vi "Func-엑셀 데이터를 그래프로 출력.vi"() -> ()   [LabVIEW 2015] (continued)
50.927\n45\t45\t50.93\n45\t45\t50.93\n45\t45\t50.933\n45\t45\t50.933\n45\t45\t50.934\n45\t45\t50.935\n45\t45\t50.93\n45\t45\t50.929\n45\t45\t50.927\n45\t45\t50.927\n45\t45\t50.927\n45\t45\t50.926\n45\t45\t50.929\n45\t45\t50.935\n45\t45\t50.938\n45\t45\t50.937\n45\t45\t50.939\n45\t45\t50.942\n45\t45\t50.94\n45\t45\t50.939\n45\t45\t50.937\n45\t45\t50.945\n45\t45\t50.944\n45\t45\t50.944\n45\t45\t50.949\n45\t45\t50.95\n45\t45\t50.952\n45\t45\t50.949\n45\t45\t50.95\n45\t45\t50.949\n45\t45\t50.95\n45\t45\t50.95\n45\t45\t50.95\n45.083\t45.06\t51.454\n45.167\t45.12\t51.454\n45.25\t44.98\t51.464\n45.333\t44.93\t51.459\n45.417\t44.88\t51.464\n45.5\t44.82\t51.465\n45.583\t44.73\t51.473\n45.667\t44.67\t51.468\n45.75\t44.61\t51.472\n45.833\t44.54\t51.482\n45.917\t44.49\t51.481\n46\t44.45\t51.484\n46.083\t44.44\t51.485\n46.167\t44.44\t51.489\n46.25\t44.46\t51.483\n46.333\t44.51\t51.48\n46.417\t44.56\t51.492\n46.5\t44.64\t51.481\n46.583\t44.72\t51.489\n46.667\t44.81\t51.487\n46.75\t44.91\t51.487\n46.833\t45.01\t51.496\n46.917\t45.11\t51.491\n47\t45.22\t51.492\n47.083\t45.34\t51.484\n47.167\t45.46\t51.488\n47.25\t45.57\t51.495\n47.333\t45.67\t51.494\n47.417\t45.78\t51.486\n47.5\t45.88\t51.496\n47.583\t45.98\t51.486\n47.667\t46.07\t51.493\n47.75\t46.16\t51.49\n47.833\t46.25\t51.499\n47.917\t46.34\t51.495\n48\t46.42\t51.504\n48.083\t46.51\t51.499\n48.167\t46.59\t51.522\n48.25\t46.67\t51.518\n48.333\t46.77\t51.516\n48.417\t46.84\t51.523\n48.5\t46.93\t51.53\n48.583\t47.01\t51.538\n48.667\t47.1\t51.536\n48.75\t47.17\t51.552\n48.833\t47.24\t51.558\n48.917\t47.32\t51.562\n49\t47.4\t51.574\n49.083\t47.48\t51.588\n49.167\t47.55\t51.587\n49.25\t47.63\t51.607\n49.333\t47.71\t51.613\n49.417\t47.79\t51.635\n49.5\t47.87\t51.639\n49.583\t47.95\t51.655\n49.667\t48.03\t51.664\n49.75\t48.11\t51.681\n49.833\t48.18\t51.702\n49.917\t48.27\t51.708\n50\t48.35\t51.731\n50.083\t48.43\t51.746\n50.167\t48.52\t51.762\n50.25\t48.61\t51.783\n50.333\t48.69\t51.804\n50.417\t48.78\t51.823\n50.5\t48.86\t51.837\n50.583\t48.95\t51.854\n50.667\t49.02\t51.886\n50.75\t49.11\t51.9\n50.833\t49.19\t51.919\n50.917\t49.28\t51.943\n51\t49.35\t51.965\n51.083\t49.43\t51.987\n51.167\t49.52\t52.009\n51.25\t49.61\t52.038\n51.333\t49.68\t52.061\n51.417\t49.76\t52.08\n51.5\t49.83\t52.113\n51.583\t49.91\t52.137\n51.667\t49.99\t52.161\n51.75\t50.07\t52.2\n51.833\t50.15\t52.221\n51.917\t50.23\t52.246\n52\t50.31\t52.281\n52.083\t50.39\t52.312\n52.167\t50.49\t52.343\n52.25\t50.57\t52.374\n52.333\t50.65\t52.403\n52.417\t50.73\t52.438\n52.5\t50.82\t52.46\n52.583\t50.89\t52.497\n52.667\t50.98\t52.536\n52.75\t51.07\t52.575\n52.833\t51.16\t52.593\n52.917\t51.24\t52.629\n53\t51.32\t52.674\n53.083\t51.4\t52.711\n53.167\t51.48\t52.737\n53.25\t51.57\t52.782\n53.333\t51.66\t52.818\n53.417\t51.74\t52.858\n53.5\t51.82\t52.893\n53.583\t51.89\t52.931\n53.667\t51.97\t52.97\n53.75\t52.05\t53.007\n53.833\t52.14\t53.043\n53.917\t52.22\t53.093\n54\t52.3\t53.124\n54.083\t52.38\t53.176\n54.167\t52.47\t53.209\n54.25\t52.54\t53.245\n54.333\t52.64\t53.289\n54.417\t52.72\t53.343\n54.5\t52.79\t53.374\n54.583\t52.86\t53.423\n54.667\t52.94\t53.472\n54.75\t53.03\t53.514\n54.833\t53.11\t53.549\n54.917\t53.2\t53.603\n55\t53.28\t53.643\n55.083\t53.37\t53.687\n55.167\t53.44\t53.737\n55.25\t53.52\t53.783\n55.333\t53.61\t53.831\n55.417\t53.7\t53.877\n55.5\t53.78\t53.917\n55.583\t53.86\t53.972\n55.667\t53.93\t54.016\n55.75\t54.02\t54.066\n55.833\t54.1\t54.117\n55.917\t54.18\t54.164\n56\t54.27\t54.219\n56.083\t54.34\t54.265\n56.167\t54.42\t54.307\n56.25\t54.5\t54.362\n56.333\t54.58\t54.414\n56.417\t54.66\t54.463\n56.5\t54.73\t54.522\n56.583\t54.79\t54.571\n56.667\t54.88\t54.629\n56.75\t54.96\t54.674\n56.833\t55.03\t54.72\n56.917\t55.1\t54.784\n57\t55.19\t54.833\n57.083\t55.26\t54.886\n57.167\t55.34\t54.939\n57.25\t55.41\t54.992\n57.333\t55.49\t55.051\n57.417\t55.58\t55.099\n57.5\t55.66\t55.154\n57.583\t55.75\t55.209\n57.667\t55.82\t55.265\n57.75\t55.91\t55.312\n57.833\t55.99\t55.375\n57.917\t56.07\t55.438\n58\t56.16\t55.492\n58.083\t56.24\t55.546\n58.167\t56.31\t55.595\n58.25\t56.38\t55.664\n58.333\t56.47\t55.716\n58.417\t56.56\t55.777\n58.5\t56.65\t55.834\n58.583\t56.73\t55.902\n58.667\t56.8\t55.946\n58.75\t56.88\t56.002\n58.833\t56.96\t56.062\n58.917\t57.06\t56.121\n59\t57.15\t56.189\n59.083\t57.22\t56.238\n59.167\t57.3\t56.307\n59.25\t57.38\t56.354\n59.333\t57.46\t56.419\n59.417\t57.53\t56.482\n59.5\t57.61\t56.538\n59.583\t57.69\t56.598\n59.667\t57.77\t56.665\n59.75\t57.86\t56.718\n59.833\t57.94\t56.78\n59.917\t58.02\t56.843\n60\t58.1\t56.904\n60.083\t58.18\t56.961\n60.167\t58.26\t57.021\n60.25\t58.35\t57.083\n60.333\t58.43\t57.157\n60.417\t58.51\t57.206\n60.5\t58.59\t57.264\n60.583\t58.66\t57.339\n60.667\t58.75\t57.397\n60.75\t58.84\t57.464\n60.833\t58.93\t57.522\n60.917\t59.02\t57.582\n61\t59.1\t57.652\n61.083\t59.19\t57.711\n61.167\t59.27\t57.785\n61.25\t59.35\t57.839\n61.333\t59.45\t57.91\n61.417\t59.53\t57.975\n61.5\t59.62\t58.027\n61.583\t59.72\t58.096\n61.667\t59.8\t58.163\n61.75\t59.89\t58.225\n61.833\t59.97\t58.293\n61.917\t60.05\t58.357\n62\t60.14\t58.418\n62.083\t60.22\t58.486\n62.167\t60.3\t58.55\n62.25\t60.37\t58.618\n62.333\t60.45\t58.689\n62.417\t60.53\t58.754\n62.5\t60.6\t58.819\n62.583\t60.69\t58.891\n62.667\t60.76\t58.95\n62.75\t60.84\t59.013\n62.833\t60.92\t59.083\n62.917\t61.01\t59.146\n63\t61.09\t59.214\n63.083\t61.18\t59.285\n63.167\t61.27\t59.348\n63.25\t61.35\t59.42\n63.333\t61.42\t59.478\n63.417\t61.51\t59.56\n63.5\t61.59\t59.621\n63.583\t61.68\t59.683\n63.667\t61.75\t59.76\n63.75\t61.84\t59.826\n63.833\t61.91\t59.893\n63.917\t62\t59.955\n64\t62.07\t60.034\n64.083\t62.15\t60.115\n64.167\t62.21\t60.175\n64.25\t62.3\t60.236\n64.333\t62.39\t60.311\n64.417\t62.47\t60.374\n64.5\t62.56\t60.449\n64.583\t62.65\t60.524\n64.667\t62.74\t60.598\n64.75\t62.83\t60.652\n64.833\t62.9\t60.731\n65\t62.97\t60.794\n65\t62.98\t60.795\n65\t62.99\t60.803\n65\t63\t60.809\n65\t63.01\t60.811\n65\t63.02\t60.817\n65\t63.04\t60.828\n65\t63.05\t60.836\n65\t63.05\t60.841\n65\t63.06\t60.851\n65\t63.07\t60.861\n65\t63.07\t60.867\n65\t63.08\t60.875\n65\t63.09\t60.88\n65\t63.11\t60.889\n65\t63.12\t60.898\n65\t63.13\t60.905\n65\t63.14\t60.909\n65\t63.15\t60.914\n65\t63.15\t60.922\n65\t63.16\t60.93\n65\t63.16\t60.938\n65\t63.17\t60.946\n65\t63.17\t60.953\n65\t63.18\t60.964\n65\t63.19\t60.971\n65\t63.2\t60.98\n65\t63.21\t60.988\n65\t63.22\t60.994\n65\t63.22\t61.006\n65\t63.24\t61.009\n65\t63.25\t61.012\n65\t63.26\t61.018\n65\t63.27\t61.022\n65\t63.27\t61.024\n65\t63.27\t61.031\n65\t63.28\t61.039\n65\t63.28\t61.048\n65\t63.29\t61.056\n65\t63.3\t61.064\n65\t63.31\t61.069\n65\t63.32\t61.078\n65\t63.33\t61.082\n65\t63.34\t61.088\n65\t63.35\t61.096\n65\t63.35\t61.102\n65\t63.36\t61.114\n65\t63.36\t61.121\n65\t63.37\t61.123\n65\t63.37\t61.136\n65\t63.37\t61.141\n65\t63.38\t61.146\n65\t63.39\t61.153\n65\t63.4\t61.16\n65\t63.4\t61.173\n65\t63.41\t61.178\n65\t63.42\t61.186\n65\t63.43\t61.193\n65\t63.44\t61.202\n65\t63.45\t61.209\n65\t63.45\t61.213\n65\t63.46\t61.222\n65\t63.47\t61.228\n65\t63.47\t61.234\n65\t63.47\t61.238\n65\t63.48\t61.246\n65\t63.49\t61.252\n65\t63.5\t61.26\n65\t63.51\t61.268\n65\t63.52\t61.28\n65\t63.53\t61.288\n65\t63.53\t61.292\n65\t63.54\t61.305\n65\t63.55\t61.307\n65\t63.55\t61.314\n65\t63.56\t61.32\n65\t63.57\t61.327\n65\t63.57\t61.33\n65\t63.57\t61.336\n65\t63.58\t61.346\n65\t63.59\t61.35\n65\t63.59\t61.357\n65\t63.6\t61.363\n65\t63.61\t61.375\n65\t63.61\t61.381\n65\t63.62\t61.387\n65\t63.63\t61.395\n65\t63.64\t61.401\n65\t63.64\t61.41\n65\t63.65\t61.416\n65\t63.66\t61.423\n65\t63.66\t61.429\n65\t63.67\t61.439\n65\t63.67\t61.449\n65\t63.67\t61.45\n65\t63.67\t61.455\n65\t63.68\t61.463\n65\t63.69\t61.469\n65\t63.69\t61.472\n65\t63.7\t61.477\n65\t63.71\t61.489\n65\t63.71\t61.498\n65\t63.72\t61.507\n65\t63.73\t61.509\n65\t63.74\t61.521\n65\t63.74\t61.525\n65\t63.75\t61.53\n65\t63.75\t61.535\n65\t63.76\t61.537\n65\t63.76\t61.549\n65\t63.77\t61.554\n65\t63.77\t61.56\n65\t63.77\t61.568\n65\t63.78\t61.577\n65\t63.79\t61.588\n65\t63.79\t61.605\n65\t63.8\t61.611\n65\t63.81\t61.618\n65\t63.81\t61.629\n65\t63.82\t61.635\n65\t63.83\t61.639\n65\t63.83\t61.642\n65\t63.84\t61.65\n65\t63.84\t61.654\n65\t63.85\t61.659\n65\t63.86\t61.666\n65\t63.86\t61.671\n65\t63.87\t61.679\n65\t63.87\t61.682\n65\t63.87\t61.689\n65\t63.88\t61.7\n65\t63.88\t61.709\n65\t63.89\t61.717\n65\t63.9\t61.727\n65\t63.9\t61.732\n65\t63.91\t61.739\n65\t63.91\t61.745\n65\t63.92\t61.75\n65\t63.92\t61.762\n65\t63.93\t61.763\n65\t63.93\t61.771\n65\t63.93\t61.782\n65\t63.93\t61.788\n65\t63.94\t61.795\n65\t63.94\t61.799\n65\t63.95\t61.812\n65\t63.96\t61.818\n65\t63.96\t61.827\n65\t63.97\t61.836\n65\t63.97\t61.844\n65\t63.98\t61.856\n65\t63.98\t61.862\n65\t63.98\t61.871\n65\t63.98\t61.878\n65\t63.99\t61.884\n65\t63.99\t61.889\n65\t64\t61.894\n65\t64.01\t61.898\n65\t64.01\t61.902\n65\t64.01\t61.912\n65\t64.02\t61.914\n65\t64.02\t61.922\n65\t64.03\t61.926\n65\t64.04\t61.931\n65\t64.05\t61.939\n65\t64.05\t61.948\n65\t64.06\t61.957\n65\t64.06\t61.966\n65\t64.07\t61.973\n65\t64.07\t61.982\n65\t64.08\t61.996\n65\t64.08\t62.001\n65\t64.08\t62.004\n65\t64.09\t62.016\n65\t64.1\t62.024\n65\t64.11\t62.028\n65\t64.12\t62.03\n65\t64.13\t62.035\n65\t64.13\t62.04\n65\t64.14\t62.046\n65\t64.15\t62.052\n65\t64.15\t62.062\n65\t64.16\t62.068\n65\t64.16\t62.077\n65\t64.17\t62.091\n65\t64.17\t62.094\n65\t64.18\t62.098\n65\t64.18\t62.109\n65\t64.18\t62.117\n65\t64.19\t62.121\n65\t64.19\t62.129\n65\t64.2\t62.136\n65\t64.2\t62.146\n65\t64.21\t62.152\n65\t64.21\t62.157\n65\t64.22\t62.162\n65\t64.22\t62.17\n65\t64.23\t62.176\n65\t64.23\t62.175\n65\t64.23\t62.183\n65\t64.24\t62.187\n65\t64.24\t62.195\n65\t64.24\t62.202\n65\t64.25\t62.211\n65\t64.25\t62.227\n65\t64.26\t62.232\n65\t64.26\t62.243\n65\t64.27\t62.257\n65\t64.27\t62.263\n65\t64.27\t62.268\n65\t64.28\t62.275\n65\t64.28\t62.283\n65\t64.28\t62.289\n65\t64.28\t62.296\n65\t64.29\t62.301\n65\t64.29\t62.306\n65\t64.3\t62.316\n65\t64.3\t62.325\n65\t64.31\t62.331\n65\t64.31\t62.339\n65\t64.32\t62.346\n65\t64.33\t62.353\n65\t64.33\t62.36\n65\t64.34\t62.359\n65\t64.34\t62.368\n65\t64.35\t62.374\n65\t64.35\t62.38\n65\t64.36\t62.39\n65\t64.36\t62.397\n65\t64.37\t62.405\n65\t64.37\t62.412\n65\t64.38\t62.419\n65\t64.38\t62.424\n65\t64.38\t62.43\n65\t64.38\t62.436\n65\t64.39\t62.443\n65\t64.39\t62.454\n65\t64.4\t62.459\n65\t64.4\t62.467\n65\t64.4\t62.475\n65\t64.41\t62.484\n65\t64.41\t62.491\n65\t64.42\t62.499\n65\t64.42\t62.505\n65\t64.42\t62.51\n65\t64.43\t62.521\n65\t64.44\t62.526\n65\t64.44\t62.534\n65\t64.45\t62.539\n65\t64.45\t62.545\n65\t64.45\t62.556\n65\t64.46\t62.563\n65\t64.46\t62.566\n65\t64.47\t62.575\n65\t64.47\t62.582\n65\t64.48\t62.591\n65\t64.48\t62.597\n65\t64.48\t62.602\n65\t64.49\t62.61\n65\t64.49\t62.62\n65\t64.5\t62.629\n65\t64.5\t62.632\n65\t64.51\t62.642\n65\t64.52\t62.649\n65\t64.52\t62.657\n65\t64.53\t62.662\n65\t64.53\t62.664\n65\t64.53\t62.673\n65\t64.54\t62.682\n65\t64.54\t62.689\n65\t64.55\t62.698\n65\t64.55\t62.705\n65\t64.56\t62.713\n65\t64.56\t62.718\n65\t64.57\t62.723\n65\t64.57\t62.729\n65\t64.57\t62.737\n65\t64.58\t62.74\n65\t64.58\t62.745\n65\t64.58\t62.758\n65\t64.59\t62.766\n65\t64.59\t62.769\n65\t64.59\t62.774\n65\t64.59\t62.784\n65\t64.59\t62.792\n65\t64.6\t62.798\n65\t64.6\t62.804\n65\t64.61\t62.82\n65\t64.61\t62.823\n65\t64.61\t62.827\n65\t64.62\t62.836\n65\t64.62\t62.838\n65\t64.62\t62.844\n65\t64.63\t62.85\n65\t64.63\t62.857\n65\t64.64\t62.868\n65\t64.64\t62.873\n65\t64.65\t62.882\n65\t64.65\t62.89\n65\t64.66\t62.898\n65\t64.66\t62.906\n65\t64.67\t62.913\n65\t64.67\t62.922\n65\t64.67\t62.924\n65\t64.68\t62.929\n65\t64.68\t62.934\n65\t64.68\t62.943\n65\t64.68\t62.952\n65\t64.68\t62.955\n65\t64.68\t62.966\n65\t64.69\t62.98\n65\t64.69\t62.985\n65\t64.69\t62.989\n65\t64.69\t62.998\n65\t64.69\t63.006\n65\t64.7\t63.013\n65\t64.7\t63.018\n65\t64.7\t63.025\n65\t64.71\t63.03\n65\t64.71\t63.034\n65\t64.71\t63.041\n65\t64.71\t63.051\n65\t64.72\t63.06\n65\t64.72\t63.069\n65\t64.72\t63.078\n65\t64.72\t63.086\n65\t64.73\t63.091\n65\t64.73\t63.098\n65\t64.73\t63.102\n65\t64.74\t63.108\n65\t64.74\t63.117\n65\t64.74\t63.121\n65\t64.74\t63.131\n65\t64.75\t63.135\n65\t64.75\t63.14\n65\t64.75\t63.148\n65\t64.75\t63.155\n65\t64.76\t63.164\n65\t64.76\t63.172\n65\t64.76\t63.178\n65\t64.77\t63.183\n65\t64.78\t63.188\n65\t64.78\t63.196\n65\t64.78\t63.202\n65\t64.78\t63.211\n65\t64.78\t63.217\n65\t64.78\t63.226\n65\t64.78\t63.235\n65\t64.79\t63.241\n65\t64.79\t63.249\n65\t64.79\t63.25\n65\t64.79\t63.258\n65\t64.79\t63.263\n65\t64.79\t63.268\n65\t64.79\t63.275\n65\t64.79\t63.285\n65\t64.79\t63.298\n65\t64.79\t63.305\n65\t64.79\t63.315\n65\t64.79\t63.326\n65\t64.79\t63.33\n65\t64.79\t63.337\n65\t64.79\t63.34\n65\t64.8\t63.344\n65\t64.8\t63.355\n65\t64.8\t63.36\n65\t64.8\t63.367\n65\t64.81\t63.374\n65\t64.81\t63.379\n65\t64.81\t63.386\n65\t64.82\t63.39\n65\t64.82\t63.396\n65\t64.82\t63.405\n65\t64.83\t63.408\n65\t64.83\t63.416\n65\t64.83\t63.427\n65\t64.83\t63.432\n65\t64.83\t63.439\n65\t64.83\t63.446\n65\t64.84\t63.454\n65\t64.84\t63.459\n65\t64.84\t63.465\n65\t64.84\t63.474\n65\t64.84\t63.477\n65\t64.84\t63.487\n65\t64.84\t63.495\n65\t64.85\t63.506\n65\t64.85\t63.514\n65\t64.85\t63.521\n65\t64.85\t63.53\n65\t64.85\t63.537\n65\t64.85\t63.543\n65\t64.86\t63.548\n65\t64.86\t63.553\n65\t64.86\t63.56\n65\t64.86\t63.57\n65\t64.87\t63.576\n65\t64.87\t63.58\n65\t64.87\t63.588\n65\t64.88\t63.596\n65\t64.88\t63.602\n65\t64.88\t63.607\n65\t64.88\t63.612\n65\t64.89\t63.619\n65\t64.88\t63.625\n65\t64.89\t63.631\n65\t64.89\t63.64\n65\t64.89\t63.649\n65\t64.89\t63.654\n65\t64.89\t63.662\n65\t64.89\t63.67\n65\t64.89\t63.674\n65\t64.89\t63.684\n65\t64.89\t63.689\n65\t64.9\t63.692\n65\t64.9\t63.7\n65\t64.9\t63.711\n65\t64.9\t63.717\n65\t64.9\t63.721\n65\t64.9\t63.726\n65\t64.9\t63.736\n65\t64.91\t63.742\n65\t64.9\t63.747\n65\t64.9\t63.757\n65\t64.9\t63.767\n65\t64.91\t63.772\n65\t64.92\t63.781\n65\t64.93\t63.791\n65\t64.94\t63.793\n65\t64.95\t63.802\n65\t64.96\t63.808\n65\t64.97\t63.818\n65\t64.98\t63.825\n65\t65\t63.827\n65\t64.98\t63.836\n65\t64.98\t63.839\n65\t64.98\t63.843\n65\t64.98\t63.849\n65\t64.98\t63.854\n65\t64.98\t63.859\n65\t64.98\t63.87\n65\t64.98\t63.875\n65\t64.98\t63.88\n65\t64.98\t63.891\n65\t64.98\t63.898\n65\t64.98\t63.909\n65\t64.98\t63.916\n65\t64.98\t63.922\n65\t64.98\t63.932\n65\t64.98\t63.937\n65\t64.98\t63.942\n65\t64.98\t63.946\n65\t64.98\t63.95\n65\t64.98\t63.958\n65\t64.98\t63.966\n65\t64.98\t63.974\n65\t64.98\t63.98\n65\t64.98\t63.99\n65\t64.98\t63.994\n65\t64.98\t64\n65\t64.98\t64.005\n65\t64.98\t64.01\n65\t65\t64.016\n65\t65\t64.025\n65\t65\t64.037\n65\t64.98\t64.045\n65\t65\t64.056\n65\t64.98\t64.064\n65\t65\t64.072\n65\t65\t64.075\n65\t65\t64.079\n65\t65\t64.086\n65\t65\t64.095\n65\t65\t64.101\n65\t65\t64.11\n65\t65\t64.119\n65\t65\t64.123\n65\t65\t64.127\n65\t65\t64.13\n65\t65\t64.131\n65\t65\t64.138\n65\t65\t64.145\n65\t65\t64.15\n65\t65\t64.162\n65\t65\t64.168\n65\t65\t64.176\n65\t65\t64.182\n65\t65\t64.186\n65\t65\t64.193\n65\t65\t64.199\n65\t65\t64.207\n65\t65\t64.218\n65\t65\t64.229\n65\t65\t64.234\n65\t65\t64.244\n65\t65\t64.248\n65\t65\t64.25\n65\t65\t64.258\n65\t65\t64.262\n65\t65\t64.268\n65\t65\t64.271\n65\t65\t64.278\n65\t65\t64.285\n65\t65\t64.29\n65\t65\t64.295\n65\t65\t64.299\n65\t65\t64.309\n65\t65\t64.314\n65\t65\t64.321\n65\t65\t64.325\n65\t65\t64.337\n65\t65\t64.346\n65\t65\t64.354\n65\t65\t64.357\n65\t65\t64.364\n65\t65\t64.375\n65\t65\t64.374\n65\t65\t64.378\n65\t65\t64.38\n65\t65\t64.392\n65\t65\t64.402\n65\t65\t64.405\n65\t65\t64.411\n65\t65\t64.425\n65\t65\t64.435\n65\t65\t64.438\n65\t65\t64.446\n65\t65\t64.451\n65\t65\t64.459\n65\t65\t64.465\n65\t65\t64.47\n65\t65\t64.472\n65\t65\t64.477\n65\t65\t64.483\n65\t65\t64.489\n65\t65\t64.493\n65\t65\t64.497\n65\t65\t64.511\n65\t65\t64.516\n65\t65\t64.521\n65\t65\t64.529\n65\t65\t64.534\n65\t65\t64.543\n65\t65\t64.551\n65\t65\t64.561\n65\t65\t64.576\n65\t65\t64.58\n65\t65\t64.587\n65\t65\t64.594\n65\t65\t64.599\n65\t65\t64.604\n65\t65\t64.607\n65\t65\t64.613\n65\t65\t64.617\n65\t65\t64.627\n65\t65\t64.63\n65\t65\t64.634\n65\t65\t64.647\n65\t65\t64.65\n65\t65\t64.659\n65\t65\t64.66\n65\t65\t64.665\n65\t65\t64.666\n65\t65\t64.671\n65\t65\t64.681\n65\t65\t64.692\n65\t65\t64.699\n65\t65\t64.706\n65\t65\t64.712\n65\t65\t64.714\n65\t65\t64.719\n65\t65\t64.722\n65\t65\t64.73\n65\t65\t64.738\n65\t65\t64.746\n65\t65\t64.753\n65\t65\t64.759\n65\t65\t64.766\n65\t65\t64.774\n65\t65\t64.78\n65\t65\t64.785\n65\t65\t64.787\n65\t65\t64.796\n65\t65\t64.805\n65\t65\t64.806\n65\t65\t64.815\n65\t65\t64.821\n65\t65\t64.831\n65\t65\t64.836\n65\t65\t64.839\n65\t65\t64.846\n65\t65\t64.85\n65\t65\t64.857\n65\t65\t64.867\n65\t65\t64.872\n65\t65\t64.88\n65\t65\t64.889\n65\t65\t64.898\n65\t65\t64.902\n65\t65\t64.909\n65\t65\t64.917\n65\t65\t64.922\n65\t65\t64.93\n65\t65\t64.936\n65\t65\t64.943\n65\t65\t64.95\n65\t65\t64.953\n65\t65\t64.962\n65\t65\t64.965\n65\t65\t64.97\n65\t65\t64.982\n65\t65\t64.988\n65\t65\t64.995\n65\t65\t64.998\n65\t65\t65.004\n65\t65\t65.009\n65\t65\t65.012\n65\t65\t65.014\n65\t65\t65.021\n65\t65\t65.033\n65\t65\t65.04\n65\t65\t65.046\n65\t65\t65.055\n65\t65\t65.062\n65\t65\t65.064\n65\t65\t65.067\n65\t65\t65.07\n65\t65\t65.073\n65\t65\t65.08\n65\t65\t65.083\n65\t65\t65.094\n65\t65\t65.104\n65\t65\t65.111\n65\t65\t65.122\n65\t65\t65.127\n65\t65\t65.135\n65\t65\t65.144\n65\t65\t65.146\n65\t65\t65.152\n65\t65\t65.157\n65\t65\t65.161\n65\t65\t65.165\n65\t65\t65.163\n65\t65\t65.17\n65\t65\t65.172\n65\t65\t65.176\n65\t65\t65.184\n65\t65\t65.194\n65\t65\t65.205\n65\t65\t65.208\n65\t65\t65.219\n65\t65\t65.226\n65\t65\t65.233\n65\t65\t65.241\n65\t65\t65.243\n65\t65\t65.251\n65\t65\t65.26\n65\t65\t65.264\n65\t65\t65.266\n65\t65\t65.275\n65\t65\t65.28\n65\t65\t65.286\n65\t65\t65.293\n65\t65\t65.296\n65\t65\t65.306\n65\t65\t65.307\n65\t65\t65.315\n65\t65\t65.32\n65\t65\t65.326\n65\t65\t65.331\n65\t65\t65.331\n65\t65\t65.345\n65\t65\t65.347\n65\t65\t65.357\n65\t65\t65.363\n65\t65\t65.37\n65\t65\t65.381\n65\t65\t65.381\n65\t65\t65.386\n65\t65\t65.39\n65\t65\t65.393\n65\t65\t65.4\n65\t65\t65.4\n65\t65\t65.407\n65\t65\t65.416\n65\t65\t65.422\n65\t65\t65.424\n65\t65\t65.432\n65\t65\t65.441\n65\t65\t65.445\n65\t65\t65.452\n65\t65\t65.46\n65\t65\t65.468\n65\t65\t65.475\n65\t65\t65.479\n65\t65\t65.485\n65\t65\t65.491\n65\t65\t65.494\n65\t65\t65.5\n65\t65\t65.509\n65\t65\t65.513\n65\t65\t65.517\n65\t65\t65.523\n65\t65\t65.529\n65\t65\t65.534\n65\t65\t65.534\n65\t65\t65.541\n65\t65\t65.547\n65\t65\t65.553\n65\t65\t65.559\n65\t65\t65.571\n65\t65\t65.576\n65\t65\t65.58\n65\t65\t65.585\n65\t65\t65.588\n65\t65\t65.593\n65\t65\t65.594\n65\t65\t65.598\n65\t65\t65.605\n65\t65\t65.617\n65\t65\t65.621\n65\t65\t65.627\n65\t65\t65.636\n65\t65\t65.644\n65\t65\t65.65\n65\t65\t65.656\n65\t65\t65.663\n65\t65\t65.666\n65\t65\t65.673\n65\t65\t65.679\n65\t65\t65.686\n65\t65\t65.688\n65\t65\t65.694\n65\t65\t65.702\n65\t65\t65.706\n65\t65\t65.708\n65\t65\t65.716\n65\t65\t65.718\n65\t65\t65.722\n65\t65\t65.729\n65\t65\t65.736\n65\t65\t65.742\n65\t65\t65.746\n65\t65\t65.756\n65\t65\t65.76\n65\t65\t65.763\n65\t65\t65.767\n65\t65\t65.768\n65\t65\t65.775\n65\t65\t65.778\n65\t65\t65.783\n65\t65\t65.794\n65\t65\t65.795\n65\t65\t65.802\n65\t65\t65.806\n65\t65\t65.812\n65\t65\t65.819\n65\t65\t65.824\n65\t65\t65.832\n65\t65\t65.843\n65\t65\t65.845\n65\t65\t65.848\n65\t65\t65.859\n65\t65\t65.861\n65\t65\t65.863\n65\t65\t65.87\n65\t65\t65.874\n65\t65\t65.879\n65\t65\t65.88\n65\t65\t65.886\n65\t65\t65.895\n65\t65\t65.901\n65\t65\t65.906\n65\t65\t65.912\n65\t65\t65.917\n65\t65\t65.923\n65\t65\t65.926\n65\t65\t65.93\n65\t65\t65.939\n65\t65\t65.946\n65\t65\t65.952\n65\t65\t65.958\n65\t65\t65.964\n65\t65\t65.967\n65\t65\t65.973\n65\t65\t65.98\n65\t65\t65.986\n65\t65\t65.988\n65\t65\t65.999\n65\t65\t66.007\n65\t65\t66.008\n65\t65\t66.012\n65\t65\t66.019\n65\t65\t66.029\n65\t65\t66.031\n65\t65\t66.032\n65\t65\t66.04\n65\t65\t66.046\n65\t65\t66.05\n65\t65\t66.053\n65\t65\t66.057\n65\t65\t66.062\n65\t65\t66.069\n65\t65\t66.071\n65\t65\t66.075\n65\t65\t66.086\n65\t65\t66.094\n65\t65\t66.098\n65\t65\t66.109\n65\t
